vi "getCurrentSortSearch.vi"(8 "error in (no error)":errorcluster, 11 "BasicSortedList in":refnum<class "BasicSortedList.lvclass">) -> (0 "error out":errorcluster, 2 "CurrentSortSearch":dbl, 3 "BasicSortedList out":refnum<class "BasicSortedList.lvclass">)   [LabVIEW 2010, in "BasicSortedList.lvclass"]
doc: "Gets the current number you are searching for in the sorted list."
uses:
  BasicSortedList.lvclass
  BasicSortedList.lvclass/BasicSortedList.ctl
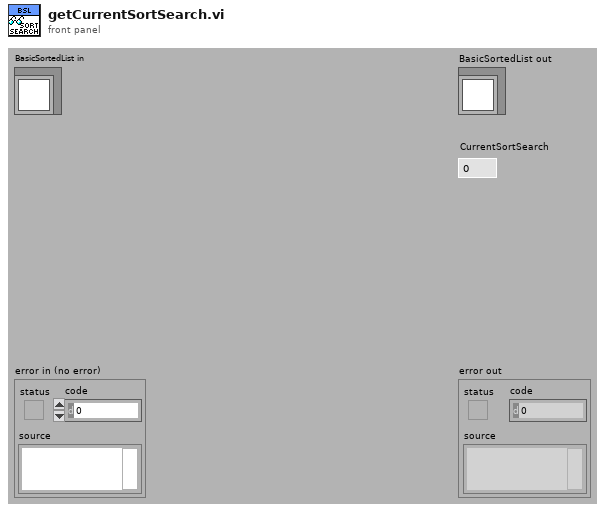
[diagram p1: front panel]
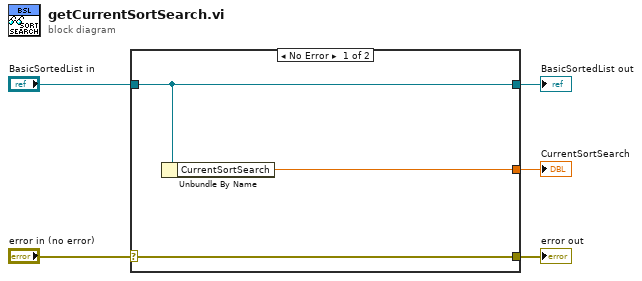
[diagram p0: block diagram]
diagram:
  n1 = case shown="No Error" "error in (no error)" {
    selector: "error in (no error)" -> [w8 w9]
    tunnel: [w8 w9] -> w4
    tunnel: [w7 w10] -> w2
    tunnel: "BasicSortedList in" -> [w7 w10]
    tunnel: [w6 _] -> w1
    frame No Error {
      n2 = Unbundle By Name(w7) -> ("CurrentSortSearch"=w6:dbl)
    }
    frame Error {
    }
  }
  "error out" <- w4
  "BasicSortedList out" <- w2
  "CurrentSortSearch" <- w1
